vi "Read Signal Samples from File.vi"() -> ()   [LabVIEW 2014]
uses:
  <vilib>/LabVIEW Universal Transcriptor/LabVIEW to Arduino Transcriptor/Transcriptors/System API/Serial println string.vi
  <vilib>/LabVIEW Universal Transcriptor/LabVIEW to Arduino Transcriptor/Transcriptors/System API/Serial print string.vi
  <vilib>/LabVIEW Universal Transcriptor/LabVIEW Universal Transcriptor SD Card Library/File.lvclass
  <vilib>/LabVIEW Universal Transcriptor/LabVIEW Universal Transcriptor SD Card Library/LabVIEW Universal Transcriptor SD Card Library.lvlib
  <vilib>/LabVIEW Universal Transcriptor/LabVIEW to Arduino Transcriptor/Transcriptors/System API/System Serial Library Variables/System Serial Library Variables.lvlib
panel:
  out "DEBUG singnal out":sgl[](graph)
  out "String Buffer":string
  out "error out":errorcluster
  in  "Error In":errorcluster
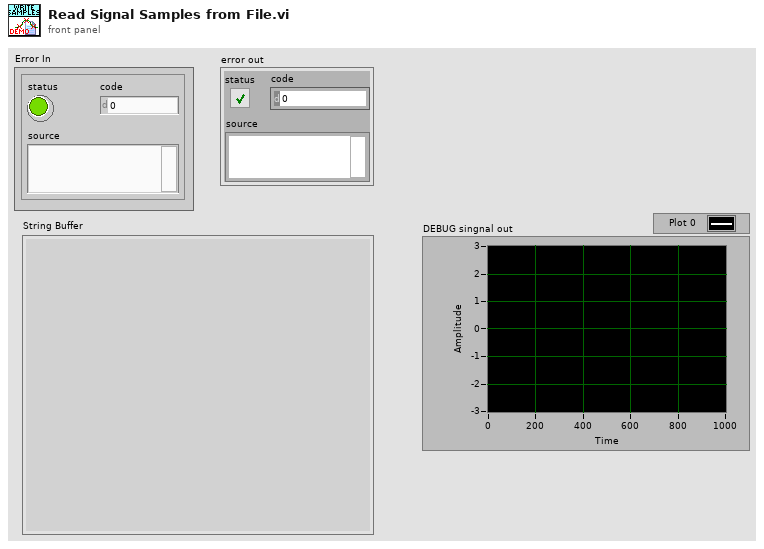
[diagram p1: front panel]
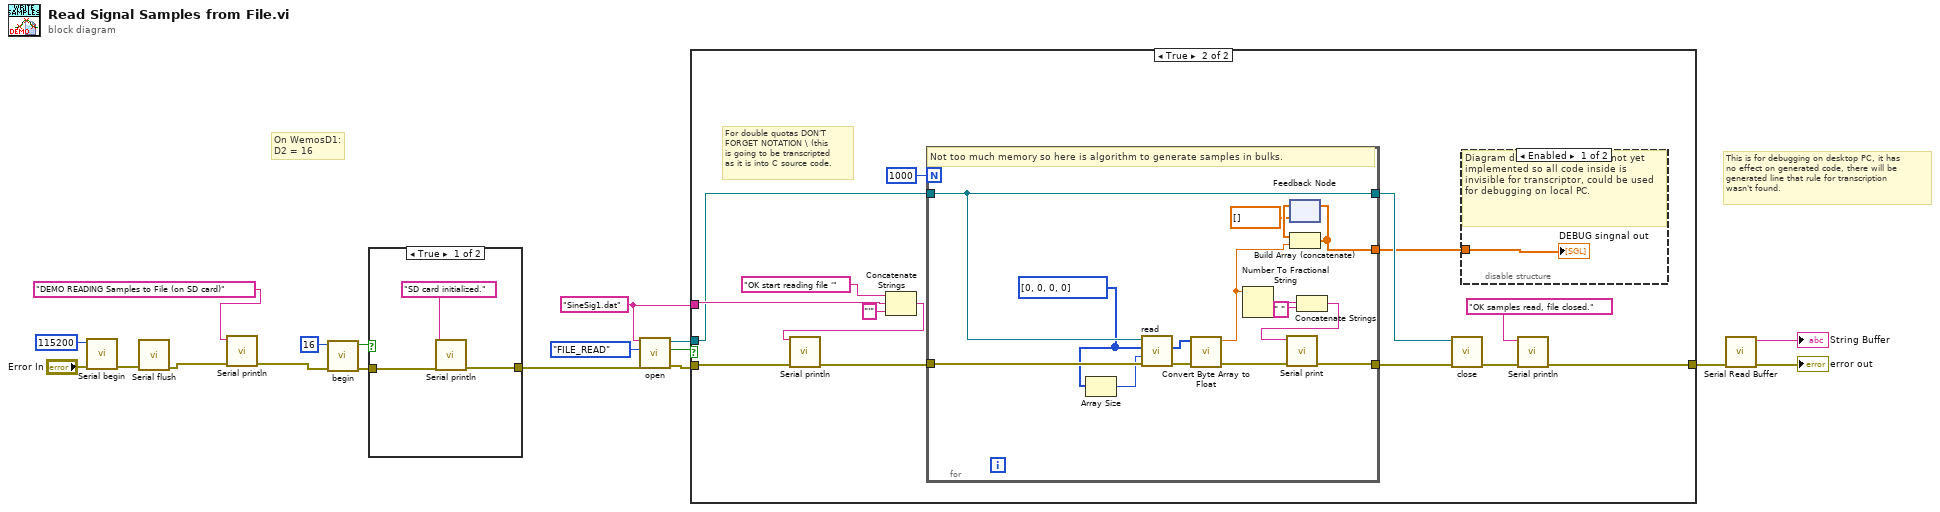
[diagram p0: block diagram]
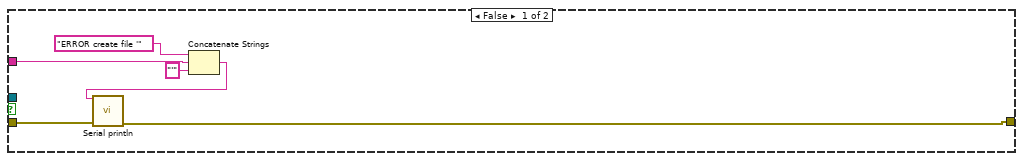
[diagram p2: hidden frame]
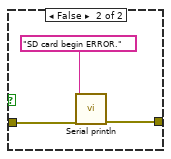
[diagram p4: hidden frame]
diagram:
  w7 = "SineSig1.dat" ("filepath")
  # "On WemosD1:\nD2 = 16"
  # "This is for debugging on desktop PC, it has\nno effect on generated code, there will be\ngenerated line that rule for transcription\nwasn't found."
  n1 = call <vilib>:"Serial begin.vi"("Error In"="Error In", "speed (Bd)"=115200) -> ("Error Out"=w18:errorcluster)  [unwired: 9 in]
  n2 = call <vilib>:"Serial flush.vi"("Error In"=w18) -> ("Error Out"=w16:errorcluster)  [unwired: 10 in]
  n3 = call-poly <vilib>:"Serial println.vi"("Error In"=w16, "string in"="DEMO READING Samples to File (on SD card)") -> ("Error Out"=w14:errorcluster)  [unwired: 9 in]
  n4 = call <vilib>:"begin.vi"("Error In"=w14, "CS pin (optional)"=u8 16) -> ("Error Out"=w11:errorcluster, "success?"=w12:bool)  [unwired: 8 in]
  n5 = case shown="True" w12 {
    tunnel: w11 -> [w21 w24]
    tunnel: [w19 w22] -> w1
    frame True {
      n6 = call-poly <vilib>:"Serial println.vi"("Error In"=w21, "string in"="SD card initialized.") -> ("Error Out"=w19:errorcluster)  [unwired: 9 in]
    }
    frame False {
      n7 = call-poly <vilib>:"Serial println.vi"("Error In"=w24, "string in"="SD card begin ERROR.") -> ("Error Out"=w22:errorcluster)  [unwired: 9 in]
    }
  }
  n8 = call <vilib>:"open.vi"("Error In"=w1, "mode"=enum16{"FILE_READ", "FILE_WRITE"}."FILE_READ", "filepath"=w7) -> ("Error Out"=w9:errorcluster, "opened?"=w8:bool, "File out"=w6:refnum<class "File.lvclass">)  [unwired: 6 in]
  n9 = case shown="True" w8 {
    tunnel: w9 -> [w26 w41]
    tunnel: w7 -> [w30 w40]
    tunnel: [w25 w33] -> w5
    tunnel: w6 -> [_ w38]
    frame False {
      n10 = Concatenate Strings("ERROR create file '" ("string in"), w30, "'" ("string")) -> (w27:string)
      n11 = call-poly <vilib>:"Serial println.vi"("Error In"=w26, "string in"=w27) -> ("Error Out"=w25:errorcluster)  [unwired: 9 in]
    }
    frame True {
      # "For double quotas DON'T\nFORGET NOTATION \\ (this\nis going to be transcripted\nas it is into C source code."
      n12 = Concatenate Strings("OK start reading file '" ("string in"), w40, "'" ("string")) -> (w42:string)
      n13 = call-poly <vilib>:"Serial println.vi"("Error In"=w41, "string in"=w42) -> ("Error Out"=w39:errorcluster)  [unwired: 9 in]
      n14 = for {
        N: 1000 -> [_]
        tunnel: w39 -> [w56]
        tunnel: w38 -> [w55]
        tunnel: [w55] -> w37
        tunnel: [w60] -> w31
        tunnel: [w46] -> w32
        w54 = u8[] [0, 0, 0, 0] ("buffer")
        # "Not too much memory so here is algorithm to generate samples in bulks."
        n15 = Array Size(array=w54) -> (size(s)=w53:i32)
        n16 = call-dynamic "read.vi"("error in (no error)"=w56, "length"=w53, "buffer"=w54, "File in"=w55) -> ("error out"=w51:errorcluster, "buffer out"=w52:u8[])  [unwired: 6 in]
        n17 = call "Convert Byte Array to Float.vi"("error in"=w51, "buffer in"=w52) -> ("error out"=w50:errorcluster, "number out"=w49:sgl)  [unwired: 8 in]
        n18 = Number To Fractional String(number=w49) -> (F-format string=w58:string)  [unwired: 3 in]
        n19 = feedback #1(sgl[] []) -> (w48:sgl[])
        n20 = Build Array (concatenate)(w48, w49) -> (w46:sgl[])
        n21 = feedback-in #1(w46) -> ()
        n22 = Concatenate Strings(w58, " " ("element")) -> (w57:string)
        n23 = call-poly <vilib>:"Serial print.vi"("Error In"=w50, "string in"=w57) -> ("Error Out"=w60:errorcluster)  [unwired: 9 in]
      }
      n24 = call-dynamic "close.vi"("error in (no error)"=w31, "File in"=w37) -> ("error out"=w34:errorcluster)  [unwired: 9 in]
      n25 = disable-structure shown="Enabled" {
        disable-tunnel: w32 -> [w45 _]
        frame Enabled {
          # "Diagram disabled structure is not yet implemented so all code inside is invisible for transcriptor, could be used for debugging on local PC."
          "DEBUG singnal out" <- w45
        }
        frame Disabled {
        }
      }
      n26 = call-poly <vilib>:"Serial println.vi"("Error In"=w34, "string in"="OK samples read, file closed.") -> ("Error Out"=w33:errorcluster)  [unwired: 9 in]
    }
  }
  n27 = call <vilib>:"Serial Read Buffer.vi"("Error In"=w5) -> ("Error Out"=→"error out":errorcluster, "String Buffer"=→"String Buffer":string)  [unwired: 9 in]
